vi "Parse Sensor Group 6.vi"(11 "stream in":u8[](array[numeric])) -> (1 "iRobot Sensor Group 6":T1={"Bumps + Wheel Drops"={"Wheeldrop Caster"=FALSE, "Wheeldrop Left"=FALSE, "Wheeldrop Right"=FALSE, "Bump Left"=FALSE, "Bump Right"=FALSE}, "Wall"=FALSE, "Cliff Left"=FALSE, "Cliff Front Left"=FALSE, "Cliff Front Right"=FALSE, "Cliff Right"=FALSE, "Wall Signal"=0, "Cliff Left Signal"=0, "Cliff Front Left Signal"=0, "Cliff Front Right Signal"=0, "Cliff Right Signal"=0, "Buttons"={"Advance"=FALSE, "Play"=FALSE}, "Virtual Wall"=FALSE, "# Stream Packets"=0, "Requested Velocity (mm/s)"=0, "Requested Radius (mm)"=0, "Requested Right Wheel Velocity (mm/s)"=0, "Requested Left Wheel Velocity (mm/s)"=0, "Distance (mm)"=0, "Angle (deg)"=0, "Song Playing"=FALSE, "Song Number"=0, "Charging State"=enum."Not Charging", "Voltage (mV)"=0, "Current (mA)"=0, "Battery Temperature (deg C)"=0, "Battery Charge (mAh)"=0, "Battery Capacity (mAh)"=0, "Charging Sources"={"Internal Charger"=FALSE, "Home Base"=FALSE}, "OI Mode"=enum."Off", "Digital Inputs"={"Digital Input 0"=FALSE, "Digital Input 1"=FALSE, "Digital Input 2"=FALSE, "Digital Input 3"=FALSE, "Device Detect"=FALSE}, "Drivers & Wheel Overcurrent"={"Low-Side Driver 0"=FALSE, "Low-Side Driver 1"=FALSE, "Low-Side Driver 2"=FALSE, "Left Wheel"=FALSE, "Right Wheel"=FALSE}, "Analog Signal"=0, "Infrared"=255} {"Infrared" format="%02x"}, 3 "stream out":u8[](array[numeric]))   [LabVIEW 2013]
doc: "Read Sensor Group 6 from a UART data stream."
uses:
  Sensor Group 6.ctl
  Bumps + Wheel Drops.ctl
  Buttons.ctl
  Charging State.ctl
  Charging Sources Available.ctl
  OI Mode.ctl
  Cargo Bay Digital Inputs.ctl
  Low-Side Driver + Wheel Overcurrent.ctl
panel:
  # "Electrical: charging, battery, OI mode"
  # "Sensors: bump, cliff, button, wheel drop, wall, virtual wall"
  # "Motion: distance, angle, requested velocity"
  # "Cargo Bay: I/O, overcurrent, infrared"
  # "Song"
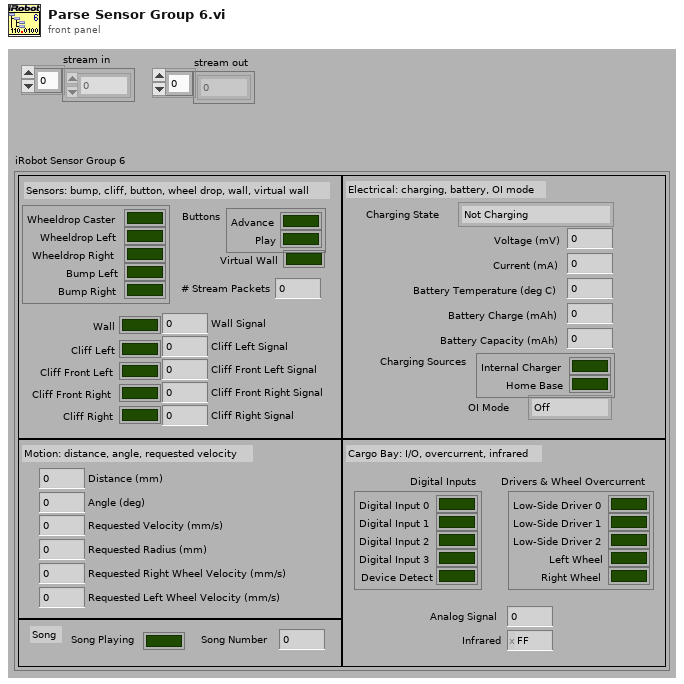
[diagram p1: front panel]
types:
  T1 = typedef "Sensor Group 6.ctl" = cluster{"Bumps + Wheel Drops":T2, "Wall":bool, "Cliff Left":bool, "Cliff Front Left":bool, "Cliff Front Right":bool, "Cliff Right":bool, "Wall Signal":u16, "Cliff Left Signal":u16, "Cliff Front Left Signal":u16, "Cliff Front Right Signal":u16, "Cliff Right Signal":u16, "Buttons":T3, "Virtual Wall":bool, "# Stream Packets":u8, "Requested Velocity (mm/s)":i16, "Requested Radius (mm)":i16, "Requested Right Wheel Velocity (mm/s)":i16, "Requested Left Wheel Velocity (mm/s)":i16, "Distance (mm)":i32, "Angle (deg)":i32, "Song Playing":bool, "Song Number":u8, "Charging State":T4, "Voltage (mV)":u16, "Current (mA)":i16, "Battery Temperature (deg C)":i8, "Battery Charge (mAh)":u16, "Battery Capacity (mAh)":u16, "Charging Sources":T5, "OI Mode":T6, "Digital Inputs":T7, "Drivers & Wheel Overcurrent":T8, "Analog Signal":u16, "Infrared":u8}
  T2 = typedef "Bumps + Wheel Drops.ctl" = cluster{"Wheeldrop Caster":bool, "Wheeldrop Left":bool, "Wheeldrop Right":bool, "Bump Left":bool, "Bump Right":bool}
  T3 = typedef "Buttons.ctl" = cluster{"Advance":bool, "Play":bool}
  T4 = typedef "Charging State.ctl" = enum16{"Not Charging", "Reconditioning Charging", "Full Charging", "Trickle Charging", "Waiting", "Charging Fault Condition"}
  T5 = typedef "Charging Sources Available.ctl" = cluster{"Internal Charger":bool, "Home Base":bool}
  T6 = typedef "OI Mode.ctl" = enum16{"Off", "Passive", "Safe", "Full"}
  T7 = typedef "Cargo Bay Digital Inputs.ctl" = cluster{"Digital Input 0":bool, "Digital Input 1":bool, "Digital Input 2":bool, "Digital Input 3":bool, "Device Detect":bool}
  T8 = typedef "Low-Side Driver + Wheel Overcurrent.ctl" = cluster{"Low-Side Driver 0":bool, "Low-Side Driver 1":bool, "Low-Side Driver 2":bool, "Left Wheel":bool, "Right Wheel":bool}
  T9 = typedef "Sensor Group 0.ctl" = cluster{"Bumps + Wheel Drops":T2, "Wall":bool, "Cliff Left":bool, "Cliff Front Left":bool, "Cliff Front Right":bool, "Cliff Right":bool, "Virtual Wall":bool, "Low-Side Driver + Wheel Overcurrent":T8, "Infrared":u8, "Buttons":T3, "Distance (mm)":i32, "Angle (deg)":i32, "Charging State":T4, "Voltage (mV)":u16, "Current (mA)":i16, "Battery Temperature (deg C)":i8, "Battery Charge (mAh)":u16, "Battery Capacity (mAh)":u16}
  T10 = typedef "Sensor Group 4.ctl" = cluster{"Wall Signal (0-4095)":u16, "Cliff Left Signal (0-4095)":u16, "Cliff Front Left Signal (0-4095)":u16, "Cliff Front Right Signal (0-4095)":u16, "Cliff Right Signal (0-4095)":u16, "Cargo Bay Digital Inputs":T7, "Cargo Bay Analog Signal (0-1023)":u16, "Charging Sources Available":T5}
  T11 = typedef "Sensor Group 5.ctl" = cluster{"OI Mode":T6, "Song Number":u8, "Song Playing":bool, "Number of Stream Packets":u8, "Requested Velocity (mm/s)":i16, "Requested Radius (mm)":i16, "Requested Right Wheel Velocity (mm/s)":i16, "Requested Left Wheel Velocity (mm/s)":i16}
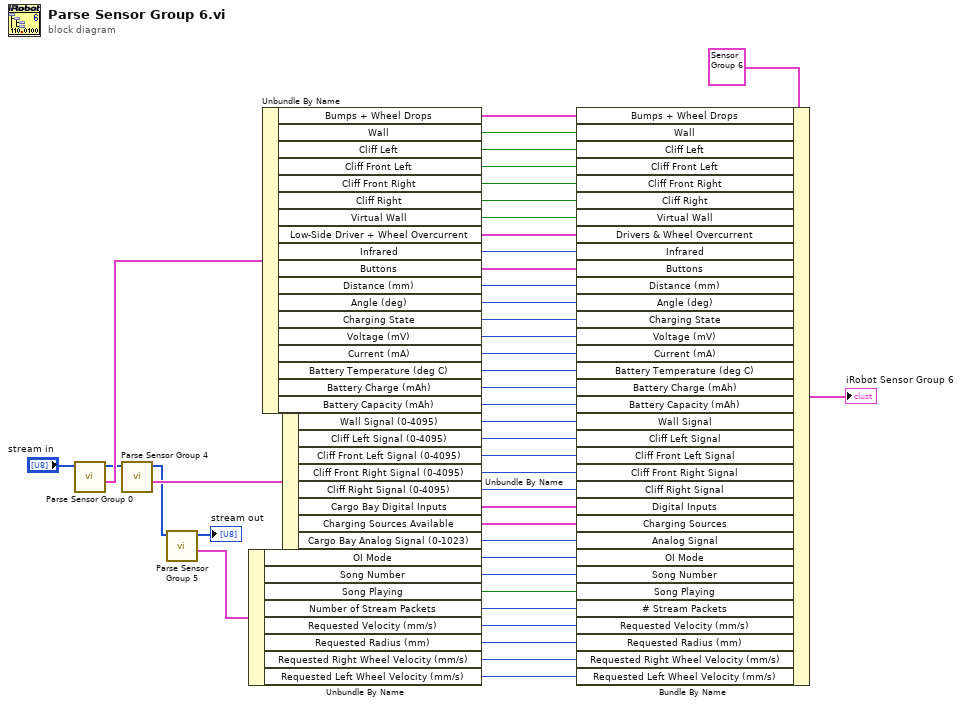
[diagram p0: block diagram]
diagram:
  n1 = call "Parse Sensor Group 0.vi"("stream in"="stream in") -> ("Sensor Group 0"=w41:T9, "stream out"=w22:u8[])  [unwired: 9 out]
  n2 = call "Parse Sensor Group 4.vi"("stream in"=w22) -> ("Sensor Group 4"=w21:T10, "stream out"=w15:u8[])  [unwired: 9 out]
  n3 = call "Parse Sensor Group 5.vi"("stream in"=w15) -> ("Sensor Group 5"=w13:T11, "stream out"=→"stream out":u8[])  [unwired: 9 out]
  n4 = Unbundle By Name(w13) -> ("OI Mode"=w9:T6, "Song Number"=w8:u8, "Song Playing"=w7:bool, "Number of Stream Packets"=w6:u8, "Requested Velocity (mm/s)"=w5:i16, "Requested Radius (mm)"=w4:i16, "Requested Right Wheel Velocity (mm/s)"=w3:i16, "Requested Left Wheel Velocity (mm/s)"=w2:i16)
  n5 = Unbundle By Name(w41) -> ("Bumps + Wheel Drops"=w40:T2, "Wall"=w39:bool, "Cliff Left"=w38:bool, "Cliff Front Left"=w37:bool, "Cliff Front Right"=w36:bool, "Cliff Right"=w35:bool, "Virtual Wall"=w34:bool, "Low-Side Driver + Wheel Overcurrent"=w33:T8, "Infrared"=w32:u8, "Buttons"=w31:T3, "Distance (mm)"=w30:i32, "Angle (deg)"=w29:i32, "Charging State"=w28:T4, "Voltage (mV)"=w27:u16, "Current (mA)"=w26:i16, "Battery Temperature (deg C)"=w25:i8, "Battery Charge (mAh)"=w24:u16, "Battery Capacity (mAh)"=w23:u16)
  n6 = Unbundle By Name(w21) -> ("Wall Signal (0-4095)"=w20:u16, "Cliff Left Signal (0-4095)"=w19:u16, "Cliff Front Left Signal (0-4095)"=w18:u16, "Cliff Front Right Signal (0-4095)"=w17:u16, "Cliff Right Signal (0-4095)"=w16:u16, "Cargo Bay Digital Inputs"=w12:T7, "Charging Sources Available"=w11:T5, "Cargo Bay Analog Signal (0-1023)"=w10:u16)
  n7 = Bundle By Name(cluster=T1 {"Bumps + Wheel Drops"={"Wheeldrop Caster"=FALSE, "Wheeldrop Left"=FALSE, "Wheeldrop Right"=FALSE, "Bump Left"=FALSE, "Bump Right"=FALSE}, "Wall"=FALSE, "Cliff Left"=FALSE, "Cliff Front Left"=FALSE, "Cliff Front Right"=FALSE, "Cliff Right"=FALSE, "Wall Signal"=0, "Cliff Left Signal"=0, "Cliff Front Left Signal"=0, "Cliff Front Right Signal"=0, "Cliff Right Signal"=0, "Buttons"={"Advance"=FALSE, "Play"=FALSE}, "Virtual Wall"=FALSE, "# Stream Packets"=0, "Requested Velocity (mm/s)"=0, "Requested Radius (mm)"=0, "Requested Right Wheel Velocity (mm/s)"=0, "Requested Left Wheel Velocity (mm/s)"=0, "Distance (mm)"=0, "Angle (deg)"=0, "Song Playing"=FALSE, "Song Number"=0, "Charging State"=enum."Not Charging", "Voltage (mV)"=0, "Current (mA)"=0, "Battery Temperature (deg C)"=0, "Battery Charge (mAh)"=0, "Battery Capacity (mAh)"=0, "Charging Sources"={"Internal Charger"=FALSE, "Home Base"=FALSE}, "OI Mode"=enum."Off", "Digital Inputs"={"Digital Input 0"=FALSE, "Digital Input 1"=FALSE, "Digital Input 2"=FALSE, "Digital Input 3"=FALSE, "Device Detect"=FALSE}, "Drivers & Wheel Overcurrent"={"Low-Side Driver 0"=FALSE, "Low-Side Driver 1"=FALSE, "Low-Side Driver 2"=FALSE, "Left Wheel"=FALSE, "Right Wheel"=FALSE}, "Analog Signal"=0, "Infrared"=0} ("iRobot Sensor Group 6"), "Bumps + Wheel Drops"=w40, "Wall"=w39, "Cliff Left"=w38, "Cliff Front Left"=w37, "Cliff Front Right"=w36, "Cliff Right"=w35, "Virtual Wall"=w34, "Drivers & Wheel Overcurrent"=w33, "Infrared"=w32, "Buttons"=w31, "Distance (mm)"=w30, "Angle (deg)"=w29, "Charging State"=w28, "Voltage (mV)"=w27, "Current (mA)"=w26, "Battery Temperature (deg C)"=w25, "Battery Charge (mAh)"=w24, "Battery Capacity (mAh)"=w23, "Wall Signal"=w20, "Cliff Left Signal"=w19, "Cliff Front Left Signal"=w18, "Cliff Front Right Signal"=w17, "Cliff Right Signal"=w16, "Digital Inputs"=w12, "Charging Sources"=w11, "Analog Signal"=w10, "OI Mode"=w9, "Song Number"=w8, "Song Playing"=w7, "# Stream Packets"=w6, "Requested Velocity (mm/s)"=w5, "Requested Radius (mm)"=w4, "Requested Right Wheel Velocity (mm/s)"=w3, "Requested Left Wheel Velocity (mm/s)"=w2) -> (→"iRobot Sensor Group 6":T1)
